vi "ShutDown SLM.vi"(8 "error in (no error)":errorcluster, 11 "SLM Parameters":T1 {"Centre X" format="%.3g"; "Centre Y" format="%.3g"}) -> (0 "error out":errorcluster)   [LabVIEW 2020]
uses:
  _controls/PCIe SLM params.ctl
  <userlib>/SLM Lib/SLM Lib.lvlib
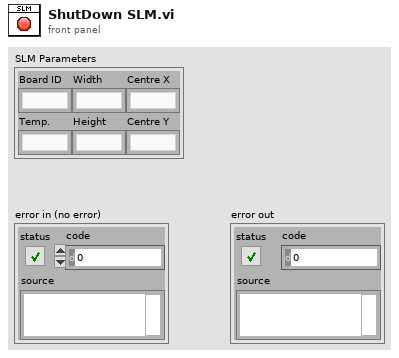
[diagram p1: front panel]
types:
  T1 = typedef "PCIe SLM params.ctl" = cluster{"Width":dbl, "Height":dbl, "Board ID":i32, "Temp.":dbl, "Centre Y":dbl, "Centre X":dbl}
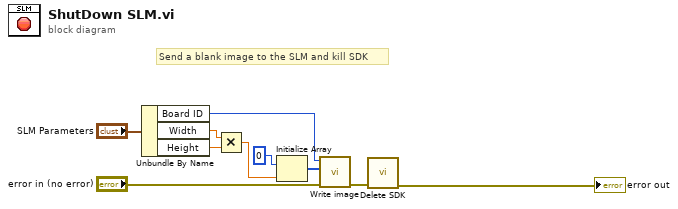
[diagram p0: block diagram]
diagram:
  # "Send a blank image to the SLM and kill SDK"
  n1 = Unbundle By Name("SLM Parameters") -> ("Board ID"=w9:i32, "Width"=w4:dbl, "Height"=w5:dbl)
  n2 = Multiply(x=w4, y=w5) -> (x*y=w6:dbl)
  n3 = Initialize Array(u8 0 ("element"), w6) -> (w8:u8[])
  n4 = call <userlib>:"Write image.vi"("error in (no error)"="error in (no error)", "image"=w8, "board"=w9) -> ("error out"=w2:errorcluster)  [unwired: 6 in, 2 out]
  n5 = call <userlib>:"Delete SDK.vi"("error in (no error)"=w2) -> ("error out"=→"error out":errorcluster)  [unwired: 10 in]
